vi "Teleop.vi"(10 "Match Info":T1={"Autonomous Elapsed Seconds"=0.0, "TeleOp Elapsed Seconds"=0.0, "Disabled Elapsed Seconds"=0.0, "Visited Autonomous"=FALSE, "Visited TeleOp"=FALSE, "Visited Disabled"=FALSE, "Autonomous Settings"={"Autonomous Style"=enum."Independent", "VI Refnum"=refnum}}, 11 "Call Context":T2) -> ()   [LabVIEW 2016]
doc: "This VI is called for each TeleOp packet received from the DS where the robot is not disabled. It is often used to read from the joysticks and update I/O or to update setpoints for timed control loops. It should complete and return within 20 milliseconds or it may miss DS packets."
uses:
  <vilib>/Rock Robotics/WPI/DriverStation/WPI_DriverStationDerivedRobotMode.ctl
  <vilib>/Rock Robotics/WPI/DriverStation/WPI_DriverStationMatch Info.ctl
  <vilib>/Rock Robotics/WPI/Solenoid/WPI_SolenoidValue.ctl
  <vilib>/Rock Robotics/WPI/Utilities/WPI_GetSetVariantRefNum.vi
  <vilib>/Rock Robotics/Network Tables/NT Read Boolean.vi
  <vilib>/Rock Robotics/Network Tables/NT Read Number.vi
  <vilib>/Rock Robotics/WPI/Solenoid/WPI_SolenoidSetEnum.vi
panel:
  out "Sample Slider 0":dbl(slide) scale=0.0..5.0
  out "Sample Boolean 1":bool
  out "Sample Boolean 0":bool
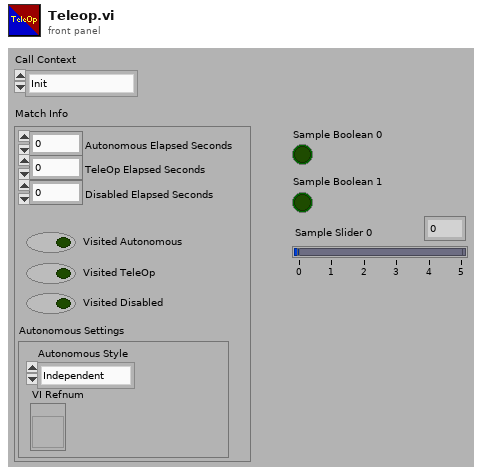
[diagram p1: front panel]
types:
  T1 = typedef "WPI_DriverStationMatch Info.ctl" = cluster{"Autonomous Elapsed Seconds":dbl, "TeleOp Elapsed Seconds":dbl, "Disabled Elapsed Seconds":dbl, "Visited Autonomous":bool, "Visited TeleOp":bool, "Visited Disabled":bool, "Autonomous Settings":cluster{"Autonomous Style":enum16{"Iterative", "Independent"}, "VI Refnum":refnum<vi>}}
  T2 = typedef "WPI_DriverStationDerivedRobotMode.ctl" = enum16{"Init", "Execute", "Stop"}
  T3 = typedef "WPI_SolenoidValue.ctl" = enum16{"Off", "On", "Forward", "Reverse"}
  T4 = typedef "WPI_JoystickDevRef.ctl" = cluster{"Device":T5}
  T5 = typedef "WPI_JoystickDeviceEnum.ctl" = enum16{"USB 0", "USB 1", "USB 2", "USB 3", "USB 4", "USB 5"}
  T6 = cluster{"Buttons[0]":bool, "Buttons[1]":bool, "Buttons[2]":bool, "Buttons[3]":bool, "Buttons[4]":bool, "Buttons[5]":bool, "Buttons[6]":bool, "Buttons[7]":bool, "Buttons[8]":bool}
  T7 = cluster{"Axes[0]":dbl, "Axes[1]":dbl, "Axes[2]":dbl, "Axes[3]":dbl, "Axes[4]":dbl, "Axes[5]":dbl, "Axes[6]":dbl, "Axes[7]":dbl, "Axes[8]":dbl}
  T8 = typedef "WPI_SolenoidDevRef.ctl" = cluster{"DevStatus":errorcluster, "Pneumatics Control Module":u8, "Forward Solenoid Channel":T9, "Reverse Solenoid Channel":T9}
  T9 = typedef "WPI_SolenoidChannel.ctl" = enum8{"Solenoid 0", "Solenoid 1", "Solenoid 2", "Solenoid 3", "Solenoid 4", "Solenoid 5", "Solenoid 6", "Solenoid 7", "Invalid"}
  T10 = typedef "WPI_RobotDriveDevRef.ctl" = cluster{"DevStatus":errorcluster, "Motors[]":T11[], "Square Inputs":bool, "Max Output":dbl}
  T11 = typedef "WPI_MotorControlDeviceRef.ctl" = cluster{"DeviceStatus":errorcluster, "Type":T12, "PWM":cluster{"PWM Channel":T13, "DeadBand":T14}, "CAN":cluster{"Device Number":u8, "SetOutput VI Ref":variant, "GetOutput VI Ref":variant, "Enable VI Ref":variant, "Disable VI Ref":variant, "Data":variant}, "Invert":bool}
  T12 = typedef "WPI_MotorControlType.ctl" = enum16{"PWM", "CAN"}
  T13 = typedef "FPGA_DIOPWMChannel.ctl" = enum8{"PWM 0", "PWM 1", "PWM 2", "PWM 3", "PWM 4", "PWM 5", "PWM 6", "PWM 7", "PWM 8", "PWM 9", "PWM MXP 0", "PWM MXP 1", "PWM MXP 2", "PWM MXP 3", "PWM MXP 4", "PWM MXP 5", "PWM MXP 6", "PWM MXP 7", "PWM MXP 8", "PWM MXP 9", "Invalid"}
  T14 = typedef "WPI_PWMDeadband.ctl" = cluster{"Name":string, "maxPositivePwm":i32, "minPositivePwm":i32, "centerPwm":i32, "maxNegativePwm":i32, "minNegativePwm":i32, "angularRange":u16}
  T15 = typedef "WPI_ServoDeviceRef.ctl" = cluster{"DeviceStatus":errorcluster, "PWM Channel":T13, "DeadBand":T14}
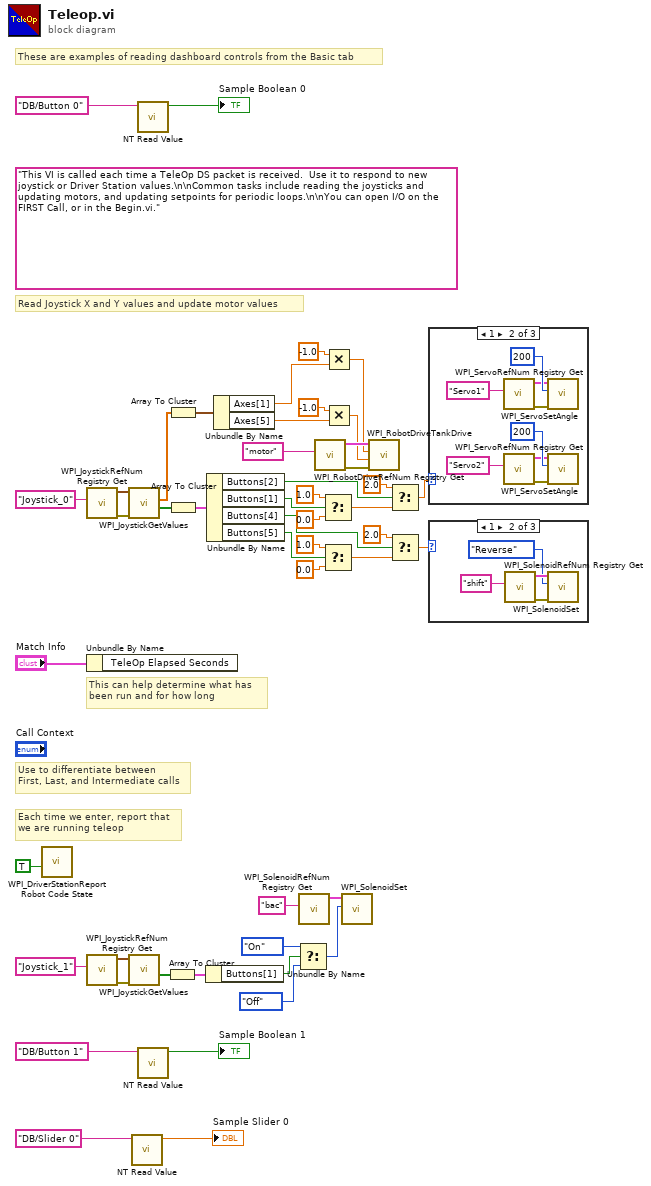
[diagram p0: block diagram]
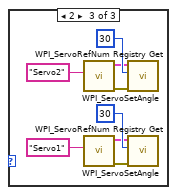
[diagram p3: hidden frame]
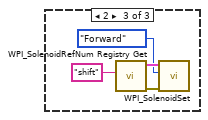
[diagram p5: hidden frame]
diagram:
  (unwired) "This VI is called each time a TeleOp DS packet is received.  Use it to respond to new joystick or Driver Station values.\n\nCommon tasks include reading the joysticks and updating motors, and updating setpoints for periodic loops.\n\nYou can open I/O on the FIRST Call, or in the Begin.vi."
  # "These are examples of reading dashboard controls from the Basic tab"
  # "Each time we enter, report that\nwe are running teleop"
  # "Use to differentiate between\nFirst, Last, and Intermediate calls"
  # "This can help determine what has\nbeen run and for how long"
  # "Read Joystick X and Y values and update motor values"
  n1 = call <vilib>:"WPI_DriverStationReport Robot Code State.vi"("TeleOp"=TRUE ("Autonomous")) -> ()  [unwired: 10 in, 1 out]
  n2 = call <vilib>:"WPI_JoystickRefNum Registry Get.vi"("refnum name"="Joystick_0") -> ("error out"=w29:errorcluster, "JoystickDevRef"=w47:T4)  [unwired: 1 in, 8 out]
  n3 = Unbundle By Name("Match Info") -> ()  [unwired: 1 out]
  n4 = call <vilib>:"WPI_JoystickRefNum Registry Get.vi"("refnum name"="Joystick_1") -> ("error out"=w28:errorcluster, "JoystickDevRef"=w30:T4)  [unwired: 1 in, 8 out]
  n5 = call <vilib>:"WPI_JoystickGetValues.vi"("error in (no error)"=w29, "JoystickDevRef"=w47) -> ("Buttons"=w38:bool[], "Axes"=w39:dbl[])  [unwired: 5 in, 3 out]
  n6 = call <vilib>:"WPI_JoystickGetValues.vi"("error in (no error)"=w28, "JoystickDevRef"=w30) -> ("Buttons"=w27:bool[])  [unwired: 5 in, 4 out]
  n7 = call-poly <vilib>:"NT Read Value.vi"("Name"="DB/Slider 0" ("refnum name")) -> ("Numeric"=→"Sample Slider 0":dbl)  [unwired: 9 in, 1 out]
  n8 = call-poly <vilib>:"NT Read Value.vi"("Name"="DB/Button 0" ("refnum name")) -> ("Boolean"=→"Sample Boolean 0":bool)  [unwired: 9 in, 1 out]
  n9 = call-poly <vilib>:"NT Read Value.vi"("Name"="DB/Button 1" ("refnum name")) -> ("Boolean"=→"Sample Boolean 1":bool)  [unwired: 9 in, 1 out]
  n10 = Array To Cluster(array=w27) -> (cluster=w26:T6)
  n11 = Array To Cluster(array=w39) -> (cluster=w37:T7)
  n12 = Array To Cluster(array=w38) -> (cluster=w36:T6)
  n13 = Unbundle By Name(w26) -> ("Buttons[1]"=w25:bool)
  n14 = Unbundle By Name(w36) -> ("Buttons[2]"=w9:bool, "Buttons[1]"=w10:bool, "Buttons[4]"=w35:bool, "Buttons[5]"=w23:bool)
  n15 = Unbundle By Name(w37) -> ("Axes[1]"=w6:dbl, "Axes[5]"=w3:dbl)
  n16 = Select(t=WPI_SolenoidValue."On" ("Value"), s=w25, f=WPI_SolenoidValue."Off" ("Value")) -> (s? t:f=w17:T3)
  n17 = call <vilib>:"WPI_SolenoidRefNum Registry Get.vi"("refnum name"="bac") -> ("SolenoidDevRef"=w18:T8)  [unwired: 9 in, 1 out]
  n18 = call <vilib>:"WPI_RobotDriveRefNum Registry Get.vi"("refnum name"="motor") -> ("error out"=w32:errorcluster, "RobotDriveDevRef"=w33:T10)  [unwired: 9 in]
  n19 = Select(t=1.0, s=w10, f=0.0) -> (s? t:f=w12:dbl)
  n20 = Select(t=1.0, s=w23, f=0.0) -> (s? t:f=w22:dbl)
  n21 = Multiply(x=-1.0, y=w6) -> (x*y=w4:dbl)
  n22 = Multiply(x=-1.0, y=w3) -> (x*y=w2:dbl)
  n23 = call-poly <vilib>:"WPI_SolenoidSet.vi"("Value"=w17, "SolenoidDevRef"=w18) -> ()  [unwired: 8 in, 2 out]
  n24 = call <vilib>:"WPI_RobotDriveTankDrive.vi"("error in (no error)"=w32, "Right axis value"=w2, "Left axis value"=w4, "RobotDriveDevRef"=w33) -> ()  [unwired: 5 in, 3 out]
  n25 = Select(t=2.0, s=w9, f=w12) -> (s? t:f=w8:dbl)
  n26 = Select(t=2.0, s=w35, f=w22) -> (s? t:f=w7:dbl)
  n27 = case shown="1" w8 {
    frame 0, Default {
    }
    frame 1 {
      n28 = call <vilib>:"WPI_ServoRefNum Registry Get.vi"("refnum name"="Servo1") -> ("error out"=w54:errorcluster, "ServoDeviceRef"=w55:T15)  [unwired: 9 in]
      n29 = call <vilib>:"WPI_ServoRefNum Registry Get.vi"("refnum name"="Servo2") -> ("error out"=w50:errorcluster, "ServoDeviceRef"=w51:T15)  [unwired: 9 in]
      n30 = call <vilib>:"WPI_ServoSetAngle.vi"("error in (no error)"=w54, "Angle"=200, "ServoDeviceRef"=w55) -> ()  [unwired: 7 in, 2 out]
      n31 = call <vilib>:"WPI_ServoSetAngle.vi"("error in (no error)"=w50, "Angle"=200, "ServoDeviceRef"=w51) -> ()  [unwired: 7 in, 2 out]
    }
    frame 2 {
      n32 = call <vilib>:"WPI_ServoRefNum Registry Get.vi"("refnum name"="Servo2") -> ("error out"=w63:errorcluster, "ServoDeviceRef"=w62:T15)  [unwired: 9 in]
      n33 = call <vilib>:"WPI_ServoRefNum Registry Get.vi"("refnum name"="Servo1") -> ("error out"=w59:errorcluster, "ServoDeviceRef"=w58:T15)  [unwired: 9 in]
      n34 = call <vilib>:"WPI_ServoSetAngle.vi"("error in (no error)"=w63, "Angle"=30, "ServoDeviceRef"=w62) -> ()  [unwired: 7 in, 2 out]
      n35 = call <vilib>:"WPI_ServoSetAngle.vi"("error in (no error)"=w59, "Angle"=30, "ServoDeviceRef"=w58) -> ()  [unwired: 7 in, 2 out]
    }
  }
  n36 = case shown="1" w7 {
    frame 0, Default {
    }
    frame 1 {
      n37 = call <vilib>:"WPI_SolenoidRefNum Registry Get.vi"("refnum name"="shift") -> ("error out"=w68:errorcluster, "SolenoidDevRef"=w67:T8)  [unwired: 9 in]
      n38 = call-poly <vilib>:"WPI_SolenoidSet.vi"("error in (no error)"=w68, "Value"=WPI_SolenoidValue."Reverse", "SolenoidDevRef"=w67) -> ()  [unwired: 7 in, 2 out]
    }
    frame 2 {
      n39 = call <vilib>:"WPI_SolenoidRefNum Registry Get.vi"("refnum name"="shift") -> ("error out"=w72:errorcluster, "SolenoidDevRef"=w71:T8)  [unwired: 9 in]
      n40 = call-poly <vilib>:"WPI_SolenoidSet.vi"("error in (no error)"=w72, "Value"=WPI_SolenoidValue."Forward", "SolenoidDevRef"=w71) -> ()  [unwired: 7 in, 2 out]
    }
  }
